vi "vesa_log_make.vi"(10 "경로와이름":string="\\vesa.log", 11 "system directory type":T1=2 items=["사용자 홈"=0, "사용자 데스크탑"=1, "사용자 문서"=2, "사용자 어플리케이션 데이터"=3, "사용자 환경"=4, "사용자 임시"=5, "퍼블릭 문서"=6, "퍼블릭 어플리케이션 데이터"=7, "퍼블릭 환경"=8, "퍼블릭 캐시"=13, "시스템 코어 라이브러리"=9, "시스템 설치된 라이브러리"=10, "어플리케이션 파일"=11, "부팅 볼륨 루트"=12]) -> (1 "Serial Port":refnum<visa-resource-name>, 3 "path":path)   [LabVIEW 2014]
uses:
  <vilib>/Utility/sysdir.llb/System Directory Type.ctl
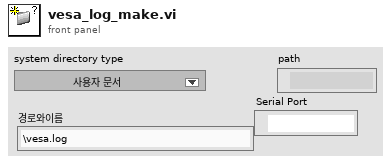
[diagram p1: front panel]
types:
  T1 = typedef "System Directory Type.ctl" = i32
  T2 = enum16{"open", "replace", "create", "open or create", "replace or create", "replace or create with confirmation"}
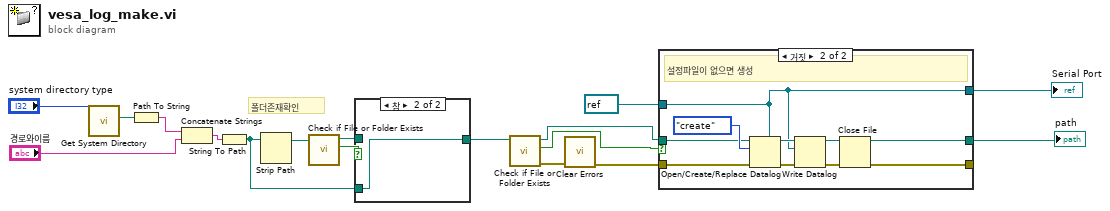
[diagram p0: block diagram]
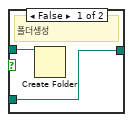
[diagram p2: hidden frame]
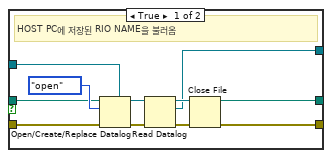
[diagram p3: hidden frame]
diagram:
  # "폴더존재확인"
  n1 = call <vilib>:"Get System Directory.vi"("system directory type"="system directory type") -> ("system directory"=w5:path)  [unwired: 10 in]
  n2 = Path To String(path=w5) -> (string=w11:string)
  n3 = Concatenate Strings(w11, "경로와이름") -> (w6:string)
  n4 = String To Path(string=w6) -> (path=w15:path)
  n5 = Strip Path(path=w15) -> (stripped path=w14:path)  [unwired: 1 out]
  n6 = call <vilib>:"Check if File or Folder Exists.vi"("path"=w14) -> ("file or folder exists?"=w12:bool, "dup path"=w13:path)  [unwired: 8 in, 1 out]
  n7 = case shown="참" w12 {
    tunnel: w13 -> [w19 _]
    tunnel: [w18 w20] -> w16
    tunnel: w15 -> [w18 w20]
    frame False {
      # "폴더생성"
      n8 = Create Folder(path (use dialog)=w19) -> ()  [unwired: 2 in, 3 out]
    }
    frame True {
    }
  }
  n9 = call <vilib>:"Check if File or Folder Exists.vi"("path"=w16) -> ("error out"=w7:errorcluster, "file or folder exists?"=w9:bool, "dup path"=w10:path)  [unwired: 8 in]
  n10 = call <vilib>:"Clear Errors.vi"("error in (no error)"=w7) -> ("error out"=w8:errorcluster)  [unwired: 5 in, 1 out]
  n11 = case shown="거짓" w9 {
    tunnel: w10 -> [w25 w33]
    tunnel: w8 -> [w26 w37]
    tunnel: refnum<visa-resource-name> refnum ("값") -> [w24 w35]
    tunnel: [w21 w35] -> w1
    tunnel: [w23 w36] -> _
    tunnel: [w22 w32] -> w17
    frame True {
      # "HOST PC에 저장된 RIO NAME을 불러옴"
      n12 = Open/Create/Replace Datalog(5:w24, 8:w26, 10:T2."open" ("동작(0:open)"), 11:w25) -> (0:w30:errorcluster, 3:w27:refnum<k1>)  [unwired: 2 in, 1 out]
      n13 = Read Datalog(4:w30, 7:w27) -> (0:w29:errorcluster, 2:w21:refnum<visa-resource-name>, 3:w28:refnum<k1>)  [unwired: 1 in]
      n14 = Close File(refnum=w28, error in=w29) -> (path=w22:path, error out=w23:errorcluster)
    }
    frame False {
      # "설정파일이 없으면 생성"
      n15 = Open/Create/Replace Datalog(5:w35, 8:w37, 10:T2."create" ("동작(0:open)"), 11:w33) -> (0:w40:errorcluster, 3:w38:refnum<k1>)  [unwired: 2 in, 1 out]
      n16 = Write Datalog(4:w40, 6:w35, 7:w38) -> (0:w39:errorcluster, 3:w34:refnum<k1>)
      n17 = Close File(refnum=w34, error in=w39) -> (path=w32:path, error out=w36:errorcluster)
    }
  }
  "path" <- w17
  "Serial Port" <- w1
